vi "Copy String Array.vi"(8 "error in":errorcluster, 9 "free (F)":bool, 10 "size":i32, 11 "pointer":i64) -> (0 "error out":errorcluster, 3 "Strings":string[](array[string]))   [LabVIEW 2020, in "G-Unicode.lvlib"]
uses:
  G-Unicode.lvlib
  4d47babd-4a2d-4eb7-b91b-7e707d692665.vi
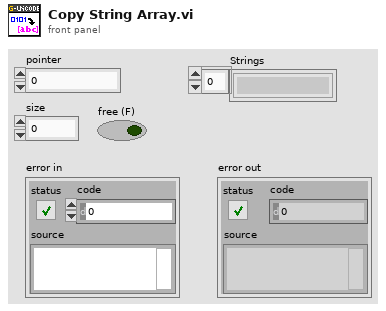
[diagram p1: front panel]
types:
  T1 = cluster{"char* string":i32, "int32_t string_length":i32}
  T2 = cluster{"char* string":i64, "int32_t string_length":i32}
  T3 = cluster{"char* string":i32, "int32_t string_length":i32}[]
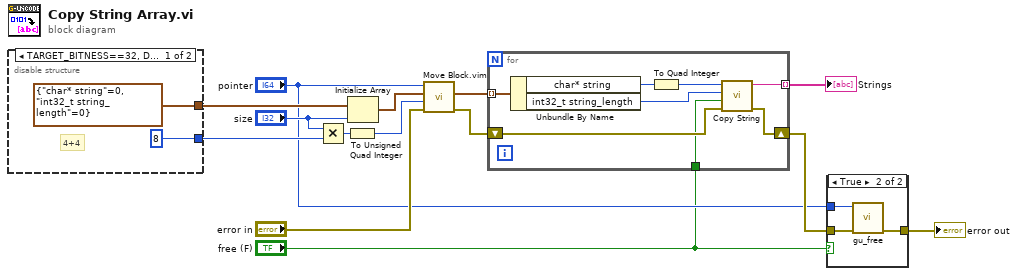
[diagram p0: block diagram]
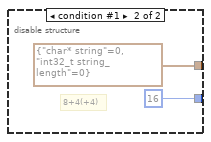
[diagram p3: hidden frame]
diagram:
  n1 = disable-structure shown="TARGET_BITNESS==32, Default" {
    disable-tunnel: [T1 {"char* string"=0, "int32_t string_length"=0} T2 {"char* string"=0, "int32_t string_length"=0}] -> w10
    disable-tunnel: [8 ("x") 16 ("x")] -> w8
    frame condition #0 (active) {
      # "4+4"
    }
    frame condition #1 {
      # "8+4(+4)"
    }
  }
  n2 = Multiply(x="size", y=w8) -> (x*y=w7:i32)
  n3 = To Unsigned Quad Integer(1:w7) -> (0:w13:u64)
  n4 = Initialize Array(w10, "size") -> (w14:T3)
  n5 = call "Move Block.vim"("error in"="error in", "memory size"=w13, "memory"=w14, "pointer"="pointer") -> ("error out"=w4:errorcluster, "filled memory"=w6:T3)  [unwired: 6 in]
  n6 = for {
    tunnel: w6 -> [w26] mode=indexing
    tunnel: [w22] -> w5 mode=indexing
    shift-right: [w20] -> w3
    shift-left: w4 -> [w21]
    tunnel: "free (F)" -> [w19]
    n7 = Unbundle By Name(w26) -> ("char* string"=w25:i32, "int32_t string_length"=w23:i32)
    n8 = To Quad Integer(1:w25) -> (0:w24:i64)
    n9 = call "Copy String.vi"("error in"=w21, "free (F)"=w19, "size"=w23, "pointer"=w24) -> ("error out"=w20:errorcluster, "string"=w22:string)  [unwired: 6 in]
  }
  "Strings" <- w5
  n10 = case shown="True" "free (F)" {
    tunnel: w3 -> [w27 w30]
    tunnel: [w27 w29] -> w11
    tunnel: "pointer" -> [_ w28]
    frame False {
    }
    frame True {
      n11 = call "gu_free.vi"("error in"=w30, "pointer"=w28) -> ("error out"=w29:errorcluster)  [unwired: 9 in]
    }
  }
  "error out" <- w11
